vi "PM-running_average.vi"(9 "Average over (10)":i32=10, 10 "new value":dbl, 11 "value array in":dbl[](array[numeric])) -> (1 "Sample size":i32, 2 "Average":dbl, 3 "value array out":dbl[](array[numeric]))   [LabVIEW 2018]
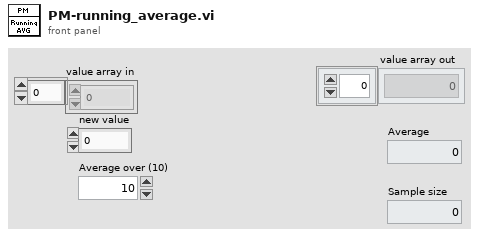
[diagram p1: front panel]
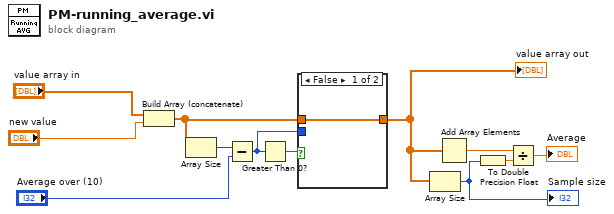
[diagram p0: block diagram]
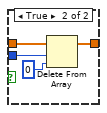
[diagram p2: hidden frame]
diagram:
  n1 = Build Array (concatenate)("value array in", "new value") -> (w9:dbl[])
  n2 = Array Size(array=w9) -> (size(s)=w12:i32)
  n3 = Subtract(x=w12, y="Average over (10)") -> (x-y=w11:i32)
  n4 = Greater Than 0?(x=w11) -> (x > 0?=w10:bool)
  n5 = case shown="False" w10 {
    tunnel: w11 -> [_ w16]
    tunnel: w9 -> [w13 w15]
    tunnel: [w13 w14] -> w5
    frame False {
    }
    frame True {
      n6 = Delete From Array(array=w15, length=w16, index=0) -> (array with subset deleted=w14:dbl[])  [unwired: 1 out]
    }
  }
  "value array out" <- w5
  n7 = Array Size(array=w5) -> (size(s)=w3:i32)
  "Sample size" <- w3
  n8 = Add Array Elements(numeric array=w5) -> (sum=w4:dbl)
  n9 = To Double Precision Float(number=w3) -> (double precision float=w2:dbl)
  n10 = Divide(x=w4, y=w2) -> (x/y=→"Average":dbl)
